vi "Strip CIDR prefix from IPv4 address.vi"(10 "prefix":i32, 11 "address U32":u32) -> (3 "address U32 out":u32)   [LabVIEW 2020, in "NI_WFCN.lvlib"]
doc: "Masks the prefix off of this address, producing the subnet address. Addresses are in native-byte-order U32 format."
uses:
  <vilib>/net/WFCN/NI_WFCN.lvlib
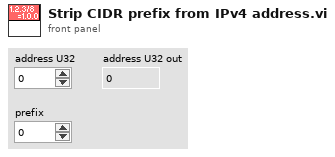
[diagram p1: front panel]
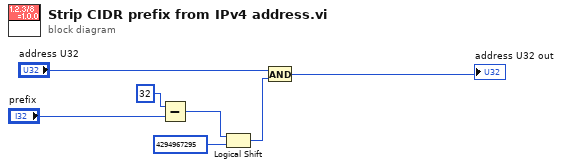
[diagram p0: block diagram]
diagram:
  n1 = Subtract(x=32, y="prefix") -> (x-y=w4:i32)
  n2 = Logical Shift(y=w4, x=u32 4294967295) -> (x << y=w5:u32)
  n3 = And(x="address U32", y=w5) -> (x .and. y?=→"address U32 out":u32)
